vi "Create_column_headers.vi"(1 "ADAM Titles":string[](array[string]), 3 "ADAM Comments":string[](array[string]), 4 "Additional Channels":string[](array[string])) -> (5 "Column headers":string[](array[string]), 6 "Header Comments":string[](array[string]), 7 "No of stats columns":i32[](array[numeric]))   [LabVIEW 2010]
uses:
  Globals/Meas_global.vi
  Globals/Dynamic_call_global.ph.vi
  Globals/LDA_meas_global_1.vi
  Acquisition/PWA/PWAtasksGLOBAL.vi
  Globals/Preference_global.vi
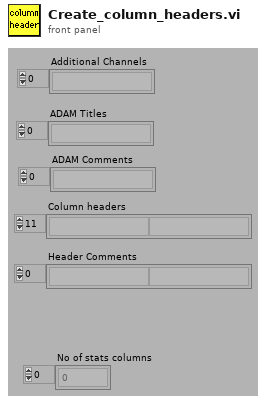
[diagram p1: front panel]
types:
  T1 = typedef "Velocity_cluster.ctl" = cluster{"Name":string, "U":dbl, "u^2":dbl, "u^3/(u^2)^(1.5)":dbl, "u^4/(u^2)^2 -3":dbl, "% u'/U":dbl, "Mean % Err":dbl, "u^4":dbl}
  T2 = typedef "PWA_Data.ctl" = enum16{"No PWA Data", "One Ch PWA"}
  T3 = typedef "Server_Comms.ctl" = enum16{"Server Link Healthy", "Do Not Link To Server"}
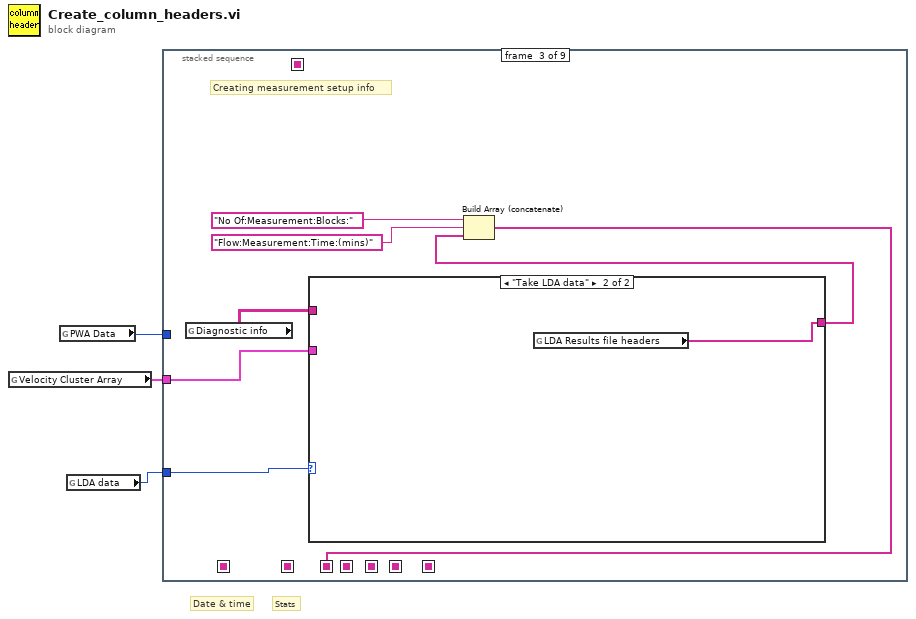
[diagram p0: block diagram]
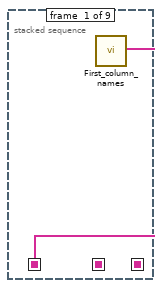
[diagram p2: hidden frame]
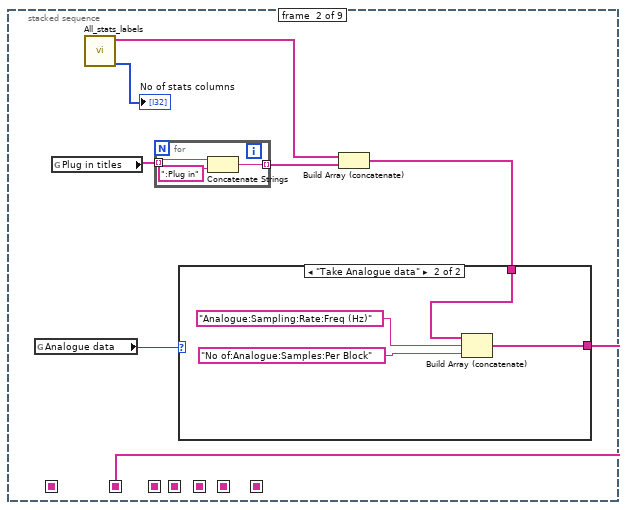
[diagram p3: hidden frame]
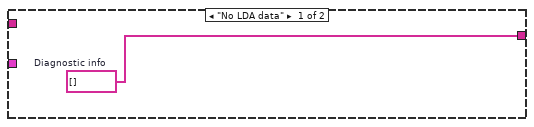
[diagram p5: hidden frame]
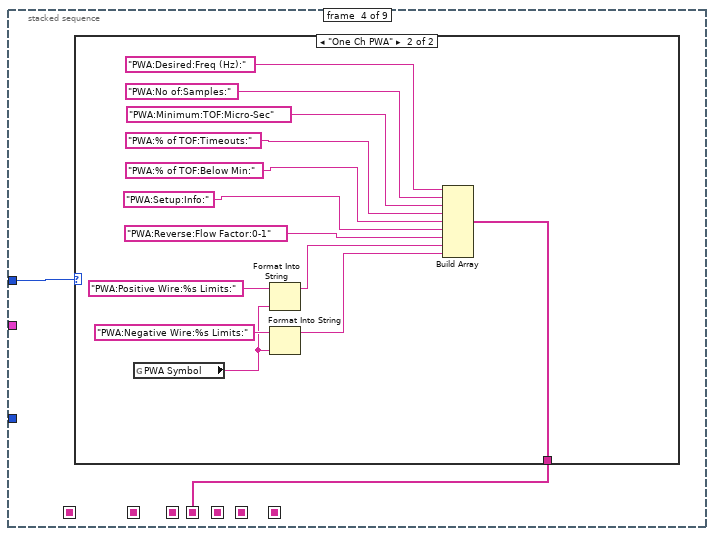
[diagram p6: hidden frame]
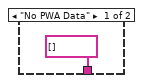
[diagram p7: hidden frame]
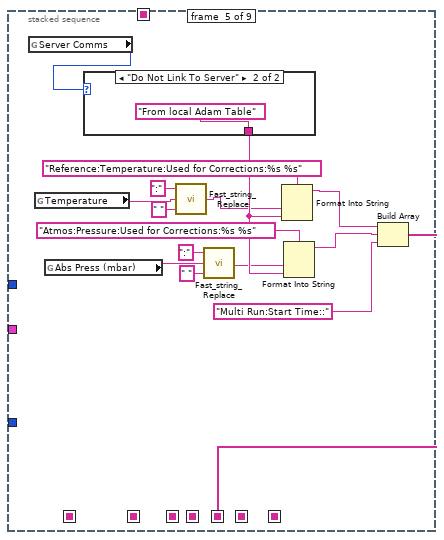
[diagram p8: hidden frame]
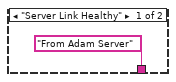
[diagram p9: hidden frame]
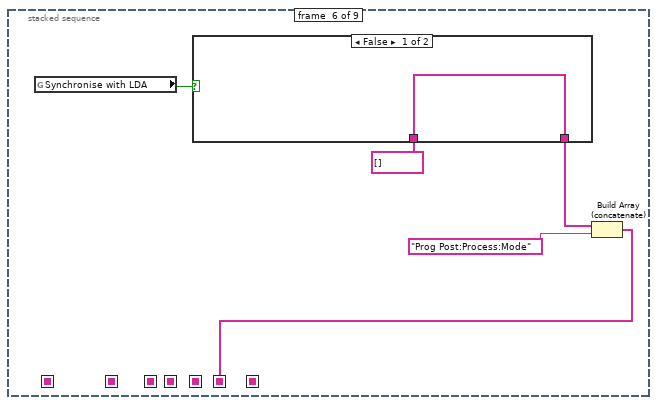
[diagram p10: hidden frame]
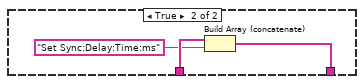
[diagram p11: hidden frame]
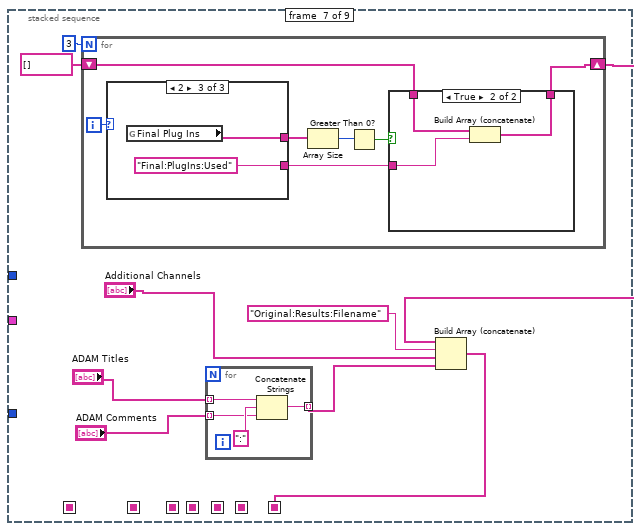
[diagram p12: hidden frame]
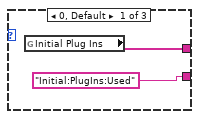
[diagram p14: hidden frame]
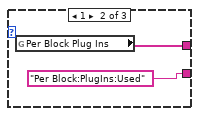
[diagram p15: hidden frame]
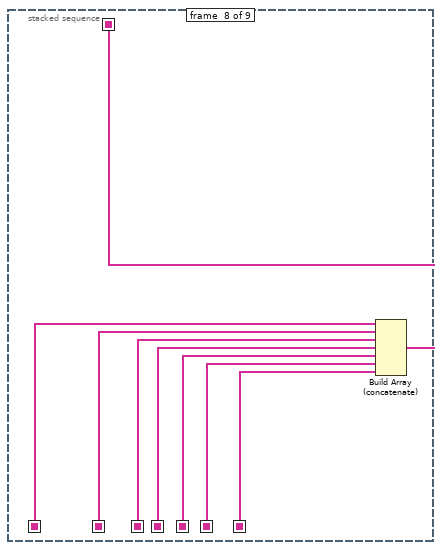
[diagram p16: hidden frame]
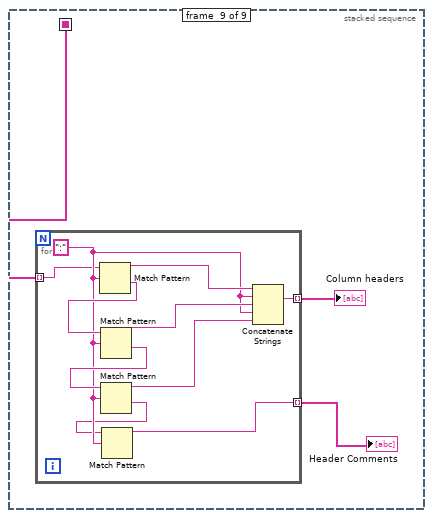
[diagram p17: hidden frame]
diagram:
  # "Stats"
  # "Date & time"
  n1 = global read "Meas_global.vi" "Velocity Cluster Array"() -> (w2:T1[])
  n2 = global read "Meas_global.vi" "PWA Data"() -> (w1:T2)
  n3 = global read "Meas_global.vi" "LDA data"() -> (w3:enum16{"No LDA data", "Take LDA data"})
  n4 = stacked-sequence {
    seq-local: [_ w5 _ _ _ _ _ _ _] -> [_ _ _ _ _ _ _ w108 _]
    seq-local: [w4 _ _ _ _ _ _ _ _] -> [_ _ _ _ _ _ _ w109 _]
    seq-local: [_ _ w24 _ _ _ _ _ _] -> [_ _ _ _ _ _ _ w107 _]
    seq-local: [_ _ _ _ _ _ w73 _ _] -> [_ _ _ _ _ _ _ w103 _]
    seq-local: [_ _ _ _ w46 _ _ _ _] -> [_ _ _ _ _ _ _ w105 _]
    seq-local: [_ _ _ _ _ _ _ w106 _] -> [_ _ _ _ _ _ _ _ w111]
    seq-local: [_ _ _ _ _ w64 _ _ _] -> [_ _ _ _ _ _ _ w104 _]
    seq-local: [_ _ _ w29 _ _ _ _ _] -> [_ _ _ _ _ _ _ w102 _]
    tunnel: w3 -> [_ _ w22 _ _ _ _ _ _]
    tunnel: w2 -> [_ _ w20 _ _ _ _ _ _]
    tunnel: w1 -> [_ _ _ w30 _ _ _ _ _]
    frame #0 {
      n5 = call "First_column_names.vi"() -> ("Array"=w4:string[])
    }
    frame #1 {
      n6 = global read "Meas_global.vi" "Analogue data"() -> (w7:enum16{"No Analogue data", "Take Analogue data"})
      n7 = global read "Dynamic_call_global.ph.vi" "Plug in titles"() -> (w10:string[])
      n8 = call "All_stats_labels.vi"() -> ("No of stats columns"=→"No of stats columns":i32[], "Stats labels"=w9:string[])  [unwired: 6 out]
      n9 = for {
        tunnel: w10 -> [w18] mode=indexing
        tunnel: [w19] -> w8 mode=indexing
        n10 = Concatenate Strings(w18, ":Plug in" ("Substring")) -> (w19:string)
      }
      n11 = Build Array (concatenate)(w9, w8) -> (w6:string[])
      n12 = case shown="\"Take Analogue data\"" w7 {
        tunnel: w6 -> [w12 w14]
        tunnel: [w12 w13] -> w5
        frame "No Analogue data" {
        }
        frame "Take Analogue data" {
          n13 = Build Array (concatenate)(w14, "Analogue:Sampling:Rate:Freq (Hz)", "No of:Analogue:Samples:Per Block") -> (w13:string[])
        }
      }
    }
    frame #2 {
      # "Creating measurement setup info"
      n14 = global read "Meas_global.vi" "Diagnostic info"() -> (w23:string[][])
      n15 = case shown="\"Take LDA data\"" w22 {
        tunnel: w23 -> [_ _]
        tunnel: [w27 w28] -> w21
        tunnel: w20 -> [_ _]
        frame "No LDA data" {
          w27 = string[] []  # Diagnostic info
        }
        frame "Take LDA data" {
          n16 = global read "LDA_meas_global_1.vi" "LDA Results file headers"() -> (w28:string[])
        }
      }
      n17 = Build Array (concatenate)("No Of:Measurement:Blocks:", "Flow:Measurement:Time:(mins)", w21) -> (w24:string[])
    }
    frame #3 {
      n18 = case shown="\"One Ch PWA\"" w30 {
        tunnel: [string[] [] w34] -> w29
        frame "No PWA Data" {
        }
        frame "One Ch PWA" {
          n19 = global read "PWAtasksGLOBAL.vi" "PWA Symbol"() -> (w42:string)
          n20 = Format Into String(format string="PWA:Positive Wire:%s Limits:", w42) -> (resulting string=w36:string)  [unwired: 2 in, 1 out]
          n21 = Format Into String(format string="PWA:Negative Wire:%s Limits:", w42) -> (resulting string=w35:string)  [unwired: 2 in, 1 out]
          n22 = Build Array("PWA:Desired:Freq (Hz):", "PWA:No of:Samples:", "PWA:Minimum:TOF:Micro-Sec", "PWA:% of TOF:Timeouts:", "PWA:% of TOF:Below Min:", "PWA:Setup:Info:", "PWA:Reverse:Flow Factor:0-1", w36, w35) -> (w34:string[])
        }
      }
    }
    frame #4 {
      n23 = global read "Preference_global.vi" "Server Comms"() -> (w60:T3)
      n24 = global read "Preference_global.vi" "Temperature"() -> (w52:string)
      n25 = global read "Preference_global.vi" "Abs Press (mbar)"() -> (w48:string)
      n26 = case shown="\"Do Not Link To Server\"" w60 {
        tunnel: ["From Adam Server" "From local Adam Table"] -> w55
        frame "Server Link Healthy" {
        }
        frame "Do Not Link To Server" {
        }
      }
      n27 = call "Fast_string_Replace.vi"("Replace match with:"=" ", "Input String"=w52, "regular expression"=":") -> ("Output String"=w51:string)  [unwired: 2 out]
      n28 = call "Fast_string_Replace.vi"("Replace match with:"=" ", "Input String"=w48, "regular expression"=":") -> ("Output String"=w47:string)  [unwired: 2 out]
      n29 = Format Into String(format string="Reference:Temperature:Used for Corrections:%s %s", w51, w55) -> (resulting string=w58:string)  [unwired: 2 in, 1 out]
      n30 = Format Into String(format string="Atmos:Pressure:Used for Corrections:%s %s", w47, w55) -> (resulting string=w56:string)  [unwired: 2 in, 1 out]
      n31 = Build Array(w58, w56, "Multi Run:Start Time::") -> (w46:string[])
    }
    frame #5 {
      n32 = global read "Meas_global.vi" "Synchronise with LDA"() -> (w67:bool)
      n33 = case shown="False" w67 {
        tunnel: [w68 w70] -> w65
        tunnel: string[] [] ("Column Titles") -> [w68 w71]
        frame False {
        }
        frame True {
          n34 = Build Array (concatenate)(w71, "Set Sync:Delay:Time:ms" ("Input Element")) -> (w70:string[])
        }
      }
      n35 = Build Array (concatenate)(w65, "Prog Post:Process:Mode" ("Input Element")) -> (w64:string[])
    }
    frame #6 {
      n36 = for {
        N: 3 -> [_]
        shift-right: [w82] -> w74
        shift-left: string[] [] -> [w83]
        i -> [w87]
        n37 = case shown="2" w87 {
          tunnel: [w93 w95 w97] -> w86
          tunnel: ["Initial:PlugIns:Used" ("Input Element") "Per Block:PlugIns:Used" ("Input Element") "Final:PlugIns:Used" ("Input Element")] -> w81
          frame 0, Default {
            n38 = global read "Dynamic_call_global.ph.vi" "Initial Plug Ins"() -> (w93:string[])
          }
          frame 1 {
            n39 = global read "Dynamic_call_global.ph.vi" "Per Block Plug Ins"() -> (w95:string[])
          }
          frame 2 {
            n40 = global read "Dynamic_call_global.ph.vi" "Final Plug Ins"() -> (w97:string[])
          }
        }
        n41 = Array Size(array=w86) -> (size(s)=w85:i32)
        n42 = Greater Than 0?(x=w85) -> (x > 0?=w84:bool)
        n43 = case shown="True" w84 {
          tunnel: w83 -> [w88 w91]
          tunnel: [w88 w90] -> w82
          tunnel: w81 -> [_ w89]
          frame False {
          }
          frame True {
            n44 = Build Array (concatenate)(w91, w89) -> (w90:string[])
          }
        }
      }
      n45 = for {
        tunnel: "ADAM Titles" -> [w100] mode=indexing
        tunnel: "ADAM Comments" -> [w99] mode=indexing
        tunnel: [w98] -> w78 mode=indexing
        n46 = Concatenate Strings(w100, ":" ("Substring"), w99) -> (w98:string)
      }
      n47 = Build Array (concatenate)(w74, "Original:Results:Filename", "Additional Channels", w78) -> (w73:string[])
    }
    frame #7 {
      n48 = Build Array (concatenate)(w109, w108, w107, w102, w105, w104, w103) -> (w106:string[])
    }
    frame #8 {
      n49 = for {
        tunnel: w111 -> [w113] mode=indexing
        tunnel: [w117] -> w110 mode=indexing
        tunnel: [w114] -> w112 mode=indexing
        w116 = ":" ("regular expression")
        n50 = Match Pattern(string=w113, regular expression=w116) -> (before substring=w120:string, after substring=w122:string)  [unwired: 3 out]
        n51 = Match Pattern(string=w122, regular expression=w116) -> (before substring=w119:string, after substring=w121:string)  [unwired: 3 out]
        n52 = Match Pattern(string=w121, regular expression=w116) -> (before substring=w118:string, after substring=w115:string)  [unwired: 3 out]
        n53 = Match Pattern(string=w115, regular expression=w116) -> (before substring=w114:string)  [unwired: 4 out]
        n54 = Concatenate Strings(w120, w116, w119, w116, w118) -> (w117:string)
      }
      "Header Comments" <- w112
      "Column headers" <- w110
    }
  }
